vi "FF_Inial.vi"() -> (3 "Array":T1[](array[typedef]))   [LabVIEW 2013]
uses:
  typeDef/AnkleTraj.ctl
  <vilib>/Analysis/baseanly.llb/Real Dot Product.vi
  <vilib>/Analysis/NI_AALBase.lvlib
panel:
  out "size(s)":i32
  in  "b FF":dbl=0.04
  in  "a FF":dbl=0.05
  in  "AnkleTraj":T1
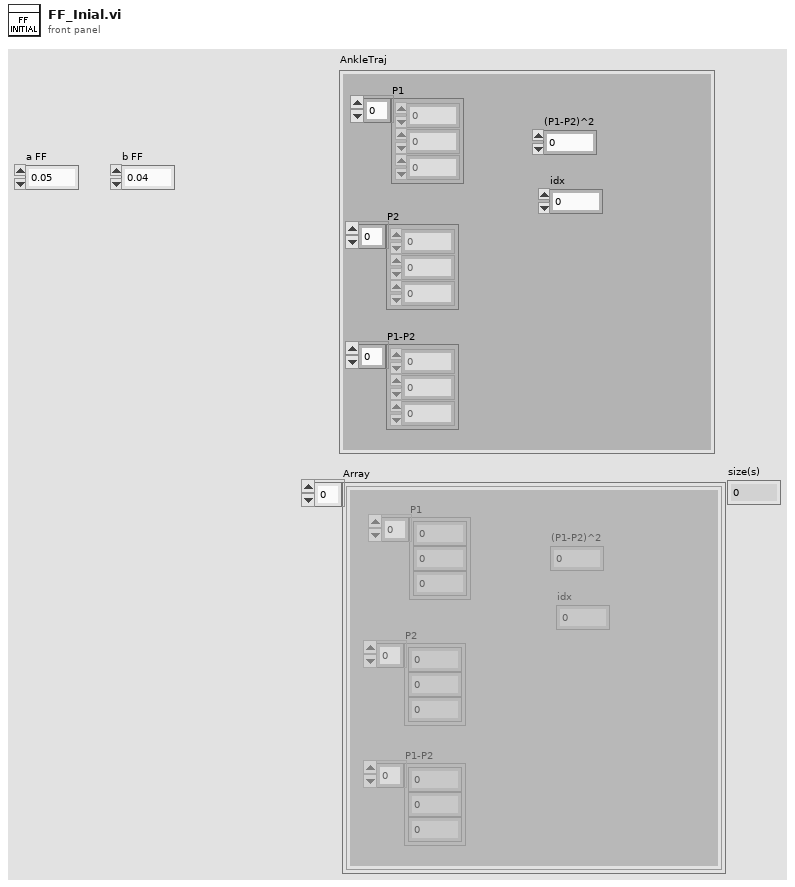
[diagram p1: front panel]
types:
  T1 = typedef "AnkleTraj.ctl" = cluster{"P1":dbl[], "P2":dbl[], "P1-P2":dbl[], "(P1-P2)^2":dbl, "idx":i32}
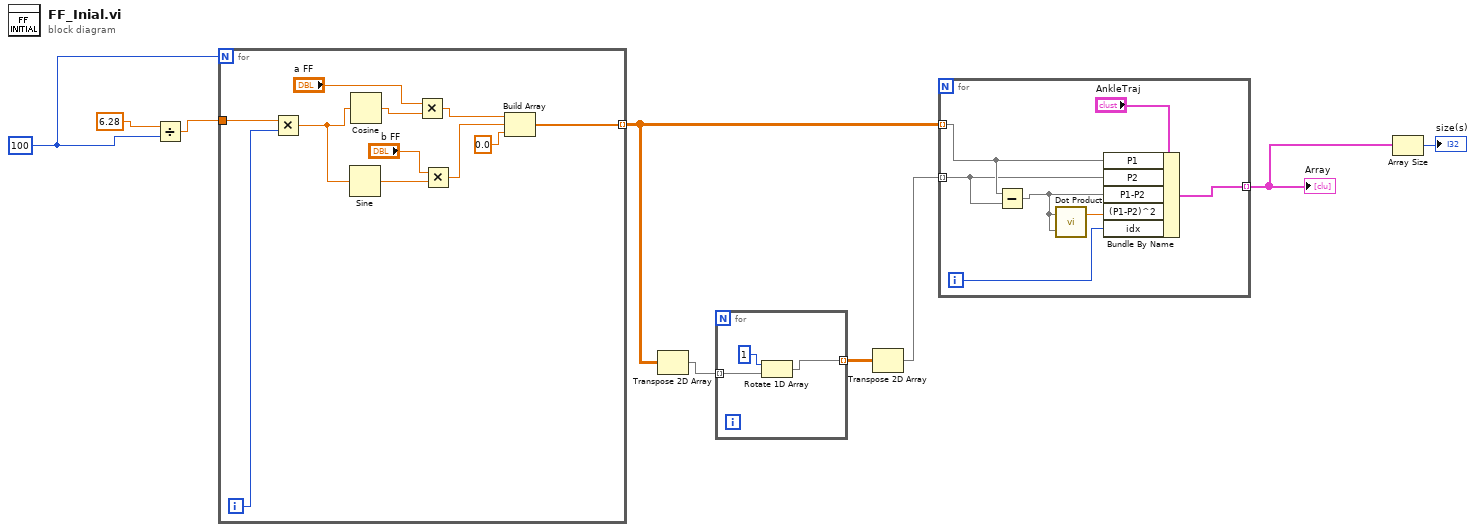
[diagram p0: block diagram]
diagram:
  w8 = 100
  n1 = Divide(x=6.28, y=w8) -> (x/y=w7:dbl)
  n2 = for {
    N: w8 -> [_]
    tunnel: w7 -> [w20]
    tunnel: [w12] -> w3 mode=indexing
    i -> [w19]
    n3 = Multiply(x=w20, y=w19) -> (x*y=w18:dbl)
    n4 = Sine(x=w18) -> (sin(x)=w16:dbl)
    n5 = Cosine(x=w18) -> (cos(x)=w17:dbl)
    n6 = Multiply(x="a FF", y=w17) -> (x*y=w15:dbl)
    n7 = Multiply(x="b FF", y=w16) -> (x*y=w14:dbl)
    n8 = Build Array(w15, w14, 0.0 ("element")) -> (w12:dbl[])
  }
  n9 = Transpose 2D Array(2D array=w3) -> (transposed array=w6:dbl[][])
  n10 = for {
    tunnel: w6 -> [w23] mode=indexing
    tunnel: [w22] -> w5 mode=indexing
    n11 = Rotate 1D Array(1:w23, 2:1 ("n")) -> (0:w22:dbl[])
  }
  n12 = Transpose 2D Array(2D array=w5) -> (transposed array=w4:dbl[][])
  n13 = for {
    tunnel: w3 -> [w29] mode=indexing
    tunnel: w4 -> [w28] mode=indexing
    tunnel: [w25] -> w2 mode=indexing
    i -> [w24]
    n14 = Subtract(x=w29, y=w28) -> (x-y=w26:dbl[])
    n15 = call-poly <vilib>:"Dot Product.vi"("Y Vector"=w26, "X Vector"=w26) -> ("X * Y"=w27:dbl)  [unwired: 1 out]
    n16 = Bundle By Name(cluster="AnkleTraj", "P1"=w29, "P2"=w28, "P1-P2"=w26, "(P1-P2)^2"=w27, "idx"=w24) -> (w25:T1)
  }
  "Array" <- w2
  n17 = Array Size(array=w2) -> (size(s)=→"size(s)":i32)
